vi "New.vi"(11 "#Samples":i32) -> (3 "VoltageMeas.lvclass":refnum<class "VoltageMeas.lvclass">)   [LabVIEW 2020, in "VoltageMeas.lvclass"]
uses:
  VoltageMeas.lvclass
  VoltageMeas.lvclass/VoltageMeas.ctl
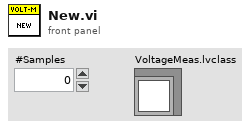
[diagram p1: front panel]
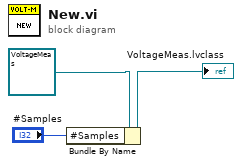
[diagram p0: block diagram]
diagram:
  n1 = Bundle By Name(cluster=refnum<class "VoltageMeas.lvclass"> refnum ("VoltageMeas.lvclass"), "#Samples"="#Samples") -> (→"VoltageMeas.lvclass":refnum<class "VoltageMeas.lvclass">)
